vi "Demo.vi"(8 "error in (no error)":errorcluster) -> ()   [LabVIEW 2012]
uses:
  DMM Base/DMM.lvclass
panel:
  out "Details":string
  out "Measurement":dbl format="%.5f"
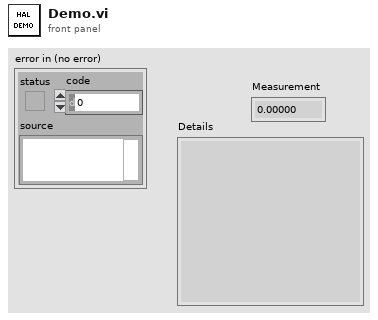
[diagram p1: front panel]
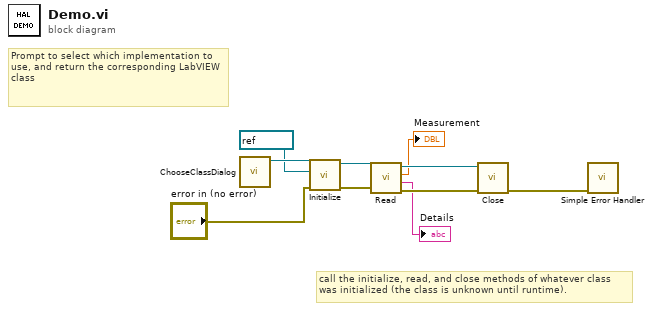
[diagram p0: block diagram]
diagram:
  # "call the initialize, read, and close methods of whatever class\nwas initialized (the class is unknown until runtime)."
  # "Prompt to select which implementation to use, and return the corresponding LabVIEW class"
  n1 = call "ChooseClassDialog.vi"() -> ("DMM out"=w6:refnum<class "DMM.lvclass">)  [unwired: 10 in, 1 out]
  n2 = call-dynamic "Initialize.vi"("error in (no error)"="error in (no error)", "Instrument Refnum in"=refnum<visa-resource-name> "Dev1", "DMM in"=w6) -> ("error out"=w3:errorcluster, "DMM out"=w5:refnum<class "DMM.lvclass">)  [unwired: 6 in, 1 out]
  n3 = call-dynamic "Read.vi"("error in (no error)"=w3, "DMM in"=w5) -> ("error out"=w9:errorcluster, "String"=→"Details":string, "Measurement"=→"Measurement":dbl, "DMM out"=w10:refnum<class "DMM.lvclass">)  [unwired: 6 in]
  n4 = call-dynamic "Close.vi"("error in (no error)"=w9, "DMM in"=w10) -> ("error out"=w7:errorcluster)  [unwired: 7 in, 2 out]
  n5 = call <vilib>:"Simple Error Handler.vi"("error in (no error)"=w7) -> ()  [unwired: 4 in, 5 out]
